vi "Is name unique.vi"(8 "error in (no error)":errorcluster, 10 "Name":string, 11 "Device Ref in":u64 format="%.0x") -> (0 "error out":errorcluster, 1 "Is name unique?":bool, 3 "Device Ref out":u64 format="%.0x")   [LabVIEW 2014, in "SLSC configuration System Explorer.lvlib"]
uses:
  SLSC configuration System Explorer.lvlib
  <vilib>/NI Veristand/Custom Device API/Custom Device API.lvlib
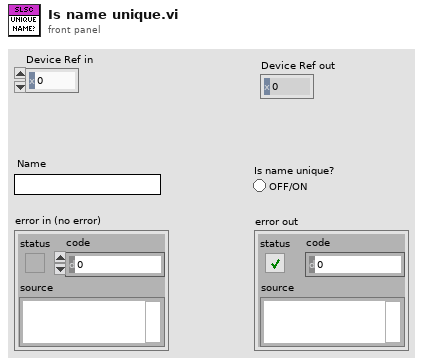
[diagram p1: front panel]
types:
  T1 = typedef "Custom Device API.lvlib/Custom Device Item Ref.ctl" = u64
  T2 = typedef "Custom Device API.lvlib/Custom Device Item Info.ctl" = cluster{"Name":string, "Is Channel":bool, "GUID":string, "Is Waveform":bool}
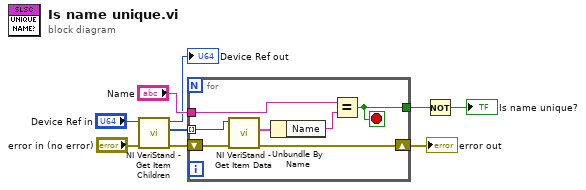
[diagram p0: block diagram]
diagram:
  n1 = call <vilib>:"NI VeriStand - Get Item Children.vi"("error in (no error)"="error in (no error)", "Item Ref in"="Device Ref in") -> ("error out"=w5:errorcluster, "Child Refs"=w3:T1[], "Item Ref out"=→"Device Ref out":T1)  [unwired: 6 in, 1 out]
  n2 = for {
    shift-right: [w13] -> w2
    shift-left: w5 -> [w10]
    tunnel: "Name" -> [w15]
    tunnel: [w12] -> w7
    tunnel: w3 -> [w11] mode=indexing
    stop <- w12 stop-if-true
    n3 = call <vilib>:"NI VeriStand - Get Item Data.vi"("error in (no error)"=w10, "Item Ref in"=w11) -> ("error out"=w13:errorcluster, "Item Info"=w16:T2)  [unwired: 8 out]
    n4 = Unbundle By Name(w16) -> ("Name"=w14:string)
    n5 = Equal?(x=w15, y=w14) -> (x = y?=w12:bool)
  }
  "error out" <- w2
  n6 = Not(x=w7) -> (.not. x?=→"Is name unique?":bool)
